vi "Create Stream Reader.vi"(8 "error in (no error)":errorcluster, 11 "Shell Stream Ref":refnum<k24>) -> (0 "error out":errorcluster, 2 "Stream Reader Ref":refnum<k24>)   [LabVIEW 2017, in "SSH.lvlib"]
uses:
  SSH.lvlib
  C:/Users/phorn/Documents/LV_SSH/Renci.SshNet.dll
  Renci.SshNet.dll
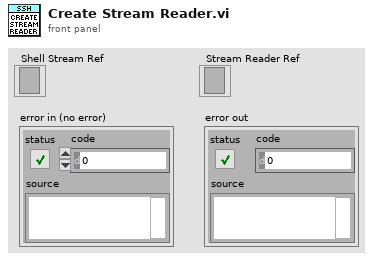
[diagram p1: front panel]
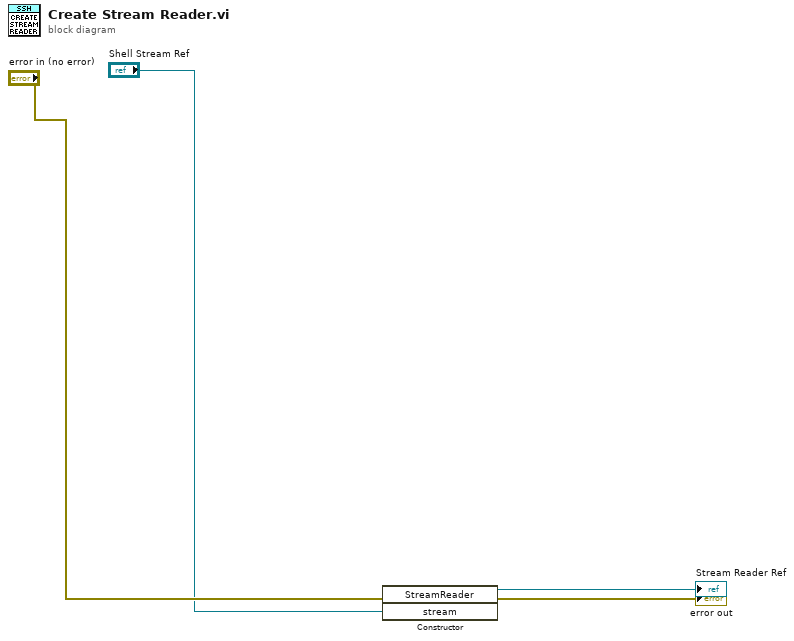
[diagram p0: block diagram]
diagram:
  n1 = constructor class="StreamReader"(error in="error in (no error)", "stream"="Shell Stream Ref") -> (reference out=→"Stream Reader Ref":refnum<k24>, error out=→"error out":errorcluster)  [unwired: 2 in, 2 out]
